vi "Common_Socket_Cmd_Sample.vi"(4 "Time Delay":i16=10, 6 "Common Socket Error in":errorcluster, 7 "Response ID 1":u8=94, 8 "Operation Message Length 1":i32=28, 9 "Operation Message ID 1":i32=93, 11 "connection ID":refnum<k5>) -> (0 "Pass":string="Horn Scan Success", 1 "error out":errorcluster, 3 "connection ID":refnum<k5>)   [LabVIEW 2017]
panel:
  out "*(type *) &x":u8
  out "rest of the binary string":string
  out "Message Length":u8
  out "Message ID":u8
  out "bytes written":i32
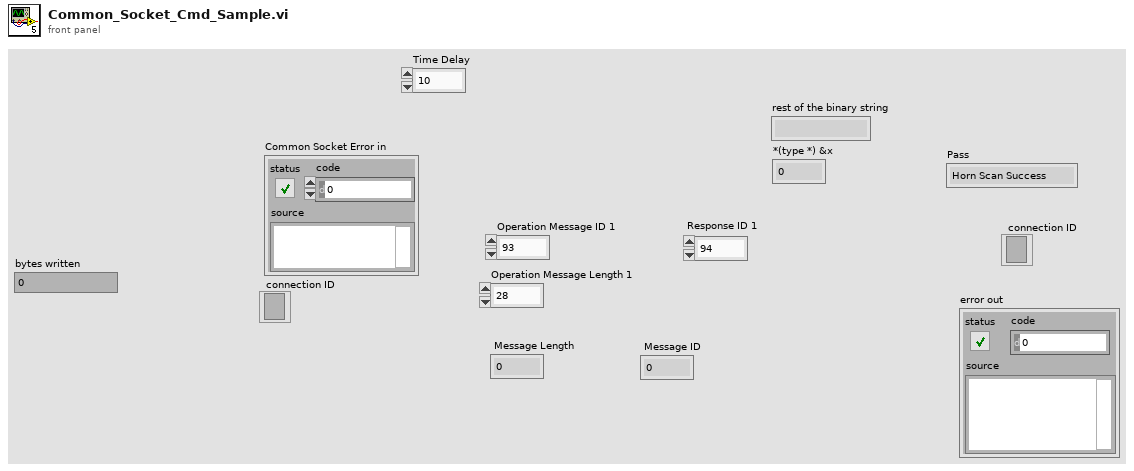
[diagram p1: front panel]
types:
  T1 = enum16{"big-endian, network order", "native, host order", "little-endian"}
  T2 = cluster{"Operation Message Length 1":i32, "Operation Message ID 1":i32}
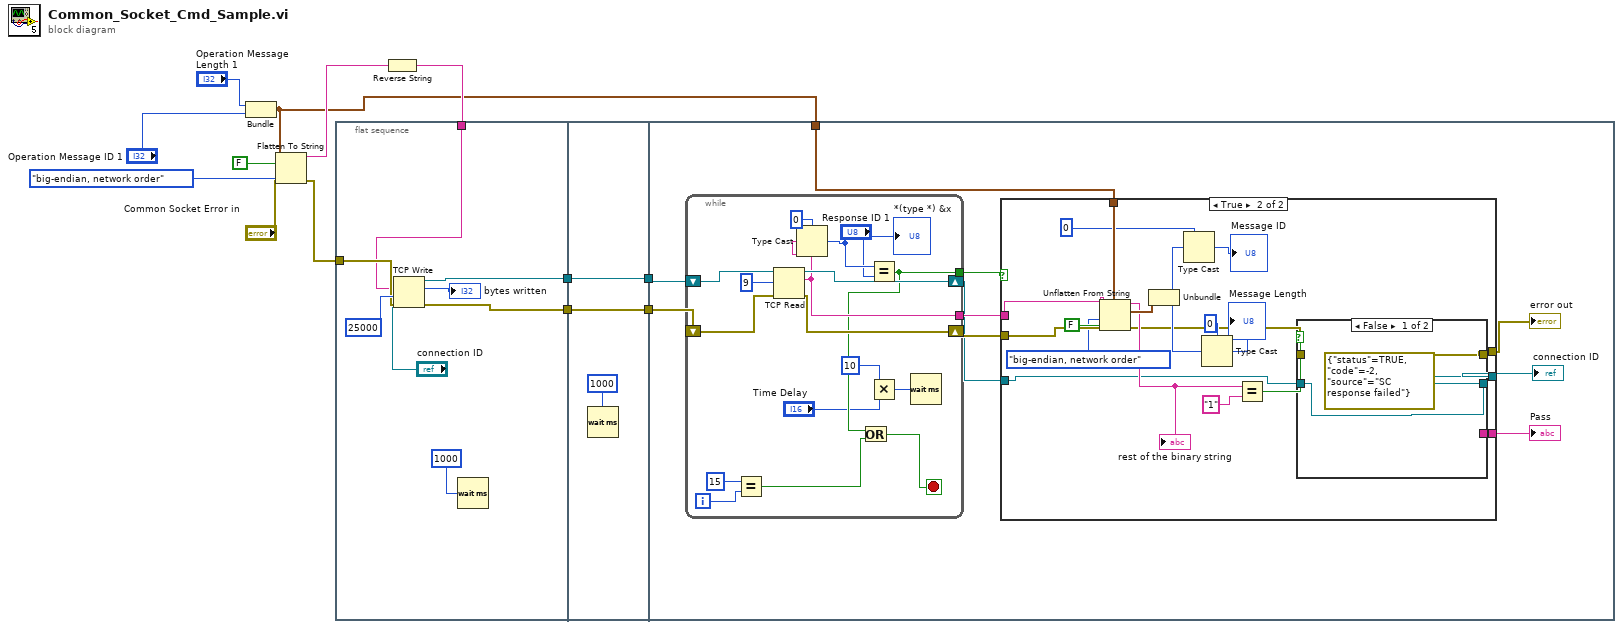
[diagram p0: block diagram]
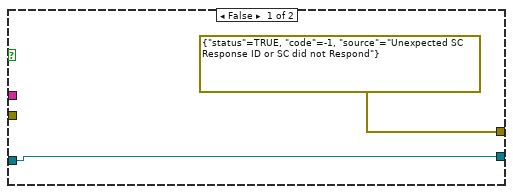
[diagram p2: hidden frame]
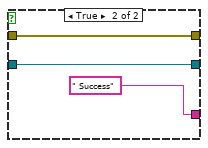
[diagram p3: hidden frame]
diagram:
  n1 = Bundle("Operation Message Length 1"="Operation Message Length 1", "Operation Message ID 1"="Operation Message ID 1") -> (w2:T2)  [unwired: 1 in]
  n2 = Flatten To String(anything=w2, prepend array or string size? (T)=FALSE, byte order (0:big-endian, network order)=T1."big-endian, network order", error in (no error)="Common Socket Error in") -> (data string=w5:string, error out=w6:errorcluster)  [unwired: 1 out]
  n3 = flat-sequence {
    tunnel: [w19] -> w13
    tunnel: [w18] -> w12
    tunnel: w6 -> [w17]
    tunnel: w4 -> [w16]
    tunnel: [w23] -> w11
    tunnel: w13 -> [w23]
    tunnel: [w22] -> w10
    tunnel: w12 -> [w22]
    tunnel: w11 -> [w34]
    tunnel: w10 -> [w33]
    tunnel: w2 -> [w32]
    frame #0 {
      n4 = TCP Write(connection ID="connection ID", data in=w16, error in (no error)=w17, 9:25000 ("timeout ms (25000)")) -> (connection ID out=w19:refnum<k5>, bytes written=→"bytes written":i32, error out=w18:errorcluster)
      n5 = Wait (ms)(milliseconds to wait=u32 1000) -> ()  [unwired: 1 out]
    }
    frame #1 {
      n6 = Wait (ms)(milliseconds to wait=u32 1000) -> ()  [unwired: 1 out]
    }
    frame #2 {
      n7 = while {
        tunnel: [w73] -> w31
        shift-right: [w76] -> w27
        shift-left: w34 -> [w78]
        shift-right: [w74] -> w30
        shift-left: w33 -> [w77]
        tunnel: [w69] -> w29
        i -> [w67]
        stop <- w68 stop-if-true
        n8 = Equal?(x=15, y=w67) -> (x = y?=w65:bool)
        n9 = TCP Read(connection ID=w78, bytes to read=9, error in (no error)=w77) -> (connection ID out=w76:refnum<k5>, data out=w73:string, error out=w74:errorcluster)  [unwired: 2 in]
        n10 = Type Cast(type=u8 0, x=w73) -> (*(type *) &x=w71:u8)
        "*(type *) &x" <- w71
        n11 = Equal?(x=w71, y="Response ID 1") -> (x = y?=w69:bool)
        n12 = Or(x=w69, y=w65) -> (x .or. y?=w68:bool)
        n13 = Multiply(x=i16 10 ("milliseconds to wait"), y="Time Delay") -> (x*y=w63:i16)
        n14 = Wait (ms)(milliseconds to wait=w63) -> ()  [unwired: 1 out]
      }
      n15 = case shown="True" w29 {
        tunnel: w32 -> [_ w55]
        tunnel: w31 -> [_ w47]
        tunnel: w30 -> [_ w46]
        tunnel: [w36 w38] -> w28
        tunnel: w27 -> [w36 w39]
        tunnel: [errorcluster {"status"=TRUE, "code"=-1, "source"="Unexpected SC Response ID or SC did not Respond"} ("error constant") w40] -> w26
        tunnel: [_ w37] -> w25
        frame False {
        }
        frame True {
          n16 = Unflatten From String(type=w55, binary string=w47, data includes array or string size? (T)=FALSE, byte order (0:big-endian, network order)=T1."big-endian, network order", error in (no error)=w46) -> (rest of the binary string=w44:string, value=w56:T2, error out=w41:errorcluster)
          "rest of the binary string" <- w44
          n17 = Unbundle(w56) -> ("Operation Message Length 1"=w49:i32, "Operation Message ID 1"=w53:i32)
          n18 = Type Cast(type=u8 0, x=w49) -> (*(type *) &x=→"Message ID":u8)
          n19 = Type Cast(type=u8 0, x=w53) -> (*(type *) &x=→"Message Length":u8)
          n20 = Equal?(x=w44, y="1") -> (x = y?=w42:bool)
          n21 = case shown="False" w42 {
            tunnel: w41 -> [_ w61]
            tunnel: [errorcluster {"status"=TRUE, "code"=-2, "source"="SC response failed"} ("error constant") w61] -> w40
            tunnel: w39 -> [w57 w60]
            tunnel: [w57 w60] -> w38
            tunnel: [_ " Success"] -> w37
            frame False {
            }
            frame True {
            }
          }
        }
      }
      "error out" <- w26
      "connection ID" <- w28
      "Pass" <- w25
    }
  }
  n22 = Reverse String(1:w5) -> (0:w4:string)
